vi "close underlying connection.vi"(8 "error in":errorcluster, 11 "connection in":refnum<class "Queue connection.lvclass">) -> (0 "error out":errorcluster)   [LabVIEW 2015, in "Queue connection.lvclass"]
uses:
  Queue connection.lvclass
  Queue connection.lvclass/Queue connection.ctl
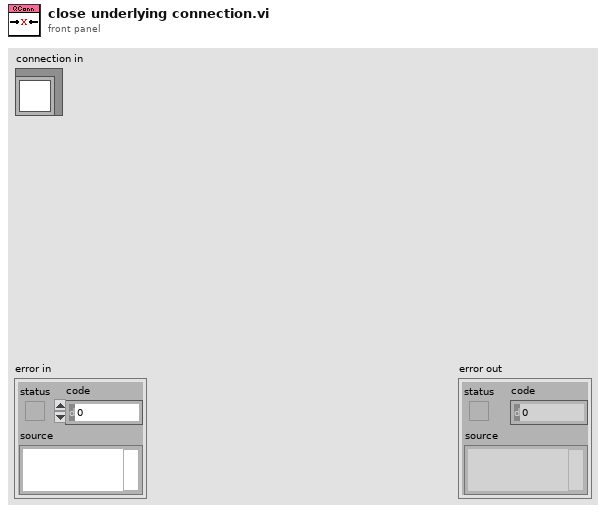
[diagram p1: front panel]
types:
  T1 = typedef "Queue connection.lvclass/queue pair.ctl" = cluster{"to pair":refnum<queue>, "from pair":refnum<queue>}
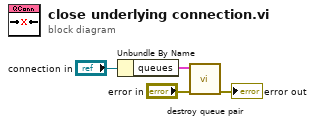
[diagram p0: block diagram]
diagram:
  n1 = Unbundle By Name("connection in") -> ("queues"=w3:T1)
  n2 = call "destroy queue pair.vi"("error in"="error in", "queue connection"=w3) -> ("error out"=→"error out":errorcluster)  [unwired: 9 in]
